vi "make_alarm_LCW.vi"(3 "enabled":bool=TRUE, 4 "WFS1_lolo":dbl=1.3, 5 "M123_lolo":dbl=0.3, 6 "WFS1_lo":dbl=1.6, 7 "M123_lo":dbl=0.6, 8 "time_last_alarm_in":timestamp, 10 "readout_status":bool=TRUE, 11 "value_array":dbl[](array[numeric])) -> (0 "time_last_alarm_out":timestamp, 2 "alarm_status":u32(colorbox))   [LabVIEW 2019]
panel:
  out "message":string
  in  "interval":dbl=600.0
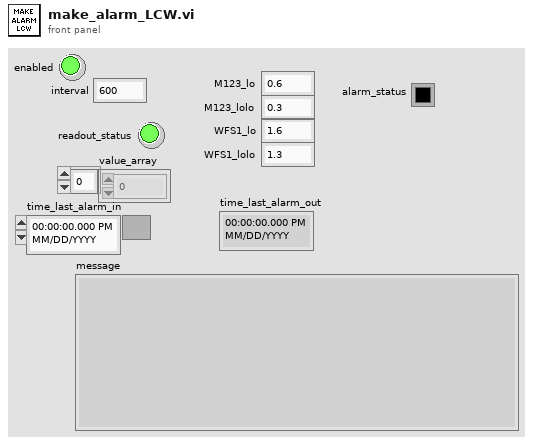
[diagram p1: front panel]
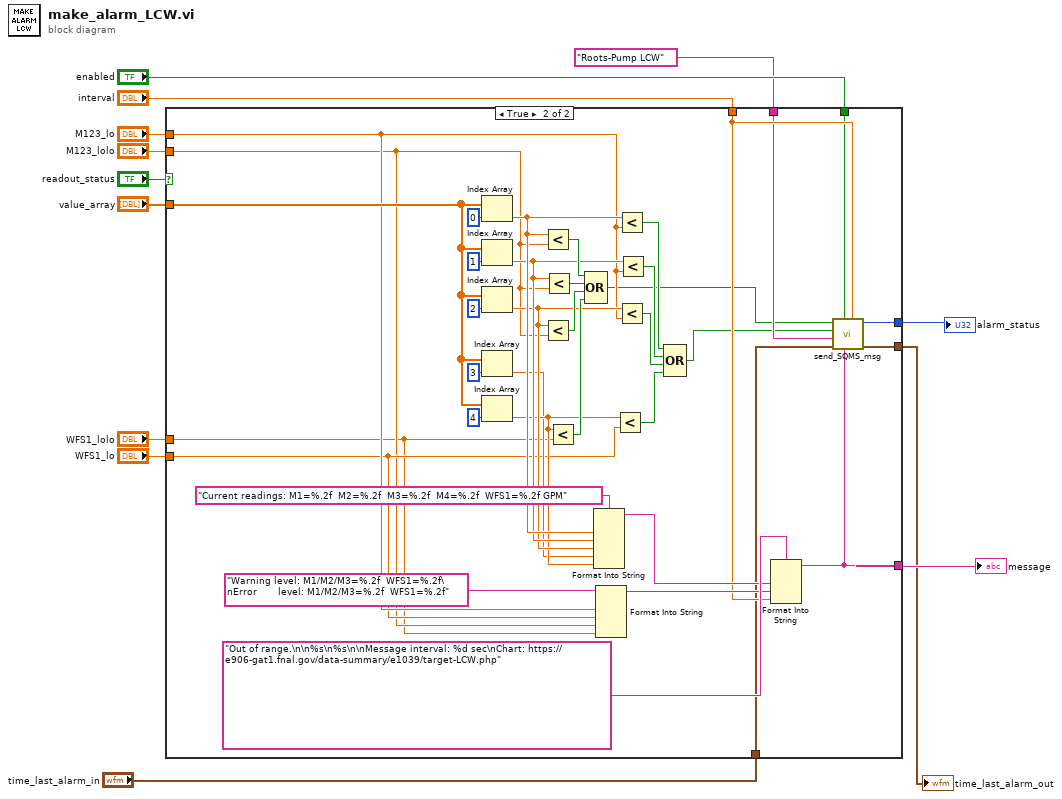
[diagram p0: block diagram]
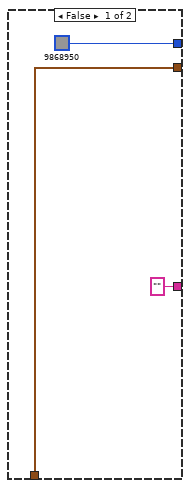
[diagram p2: hidden frame]
diagram:
  n1 = case shown="True" "readout_status" {
    tunnel: "value_array" -> [_ w40]
    tunnel: "M123_lo" -> [_ w31]
    tunnel: "WFS1_lo" -> [_ w30]
    tunnel: "M123_lolo" -> [_ w29]
    tunnel: "WFS1_lolo" -> [_ w28]
    tunnel: "interval" -> [_ w24]
    tunnel: ["" w25] -> w7
    tunnel: "enabled" -> [_ w23]
    tunnel: "time_last_alarm_in" -> [w15 w22]
    tunnel: "Roots-Pump LCW" ("title") -> [_ w21]
    tunnel: [w15 w18] -> w2
    tunnel: [u32 9868950 ("alarm_status") w17] -> w1
    frame False {
    }
    frame True {
      n2 = Index Array(array=w40, index=0) -> (element=w38:dbl)
      n3 = Index Array(array=w40, index=1) -> (element=w37:dbl)
      n4 = Index Array(array=w40, index=2) -> (element=w36:dbl)
      n5 = Index Array(array=w40, index=3) -> (element=w34:dbl)
      n6 = Index Array(array=w40, index=4) -> (element=w35:dbl)
      n7 = Less?(x=w38, y=w29) -> (x < y?=w49:bool)
      n8 = Less?(x=w36, y=w29) -> (x < y?=w47:bool)
      n9 = Less?(x=w37, y=w29) -> (x < y?=w48:bool)
      n10 = Less?(x=w35, y=w28) -> (x < y?=w46:bool)
      n11 = Compound Arithmetic op=OR(w49, w48, w47, w46) -> (w19:bool)
      n12 = Format Into String(format string="Current readings: M1=%.2f  M2=%.2f  M3=%.2f  M4=%.2f  WFS1=%.2f GPM" ("msg"), w38, w37, w36, w34, w35) -> (resulting string=w27:string)  [unwired: 2 in, 1 out]
      n13 = Format Into String(format string="Warning level: M1/M2/M3=%.2f  WFS1=%.2f\nError       level: M1/M2/M3=%.2f  WFS1=%.2f" ("msg"), w31, w30, w29, w28) -> (resulting string=w26:string)  [unwired: 2 in, 1 out]
      n14 = Less?(x=w35, y=w30) -> (x < y?=w42:bool)
      n15 = Less?(x=w38, y=w31) -> (x < y?=w45:bool)
      n16 = Less?(x=w36, y=w31) -> (x < y?=w43:bool)
      n17 = Less?(x=w37, y=w31) -> (x < y?=w44:bool)
      n18 = Compound Arithmetic op=OR(w45, w44, w43, w42) -> (w20:bool)
      n19 = Format Into String(format string="Out of range.\n\n%s\n%s\n\nMessage interval: %d sec\nChart: https://e906-gat1.fnal.gov/data-summary/e1039/target-LCW.php" ("msg"), w27, w26, w24) -> (resulting string=w25:string)  [unwired: 2 in, 1 out]
      n20 = call "send_SQMS_msg.vi"("alarm_interval"=w24, "msg"=w25, "enabled"=w23, "time_last_alarm_in"=w22, "title"=w21, "warning"=w20, "error"=w19) -> ("time_last_alarm_out"=w18:timestamp, "alarm_status"=w17:u32)  [unwired: 2 in, 1 out]
    }
  }
  "time_last_alarm_out" <- w2
  "message" <- w7
  "alarm_status" <- w1
